vi "Plot.vi"(5 "dev-Var data":dbl[](array[numeric]), 7 "Selected Variables":string[][](array[string])=[["EnergyMeter", "Channel1", "amp1", "32"], ["EnergyMeter", "Channel2", "amp2", "25"]], 9 "Currently selected items":i32[](array[numeric])) -> (4 "Plot Data":dbl[](array[numeric]))   [LabVIEW 2020]
doc: "This vi parse the configuration file data into requires to plot short term and long term plot\n[input]\n1. Selected variables\n2. Selected indices\n3. Data from TCP connection\n[output]\n1. Plot names for plot legend\n2. Plot data"
uses:
  <userlib>/_OpenG.lib/array/array.llb/Index 1D Array Elements (DBL)__ogtk.vi
panel:
  out "References":string[](array[string])
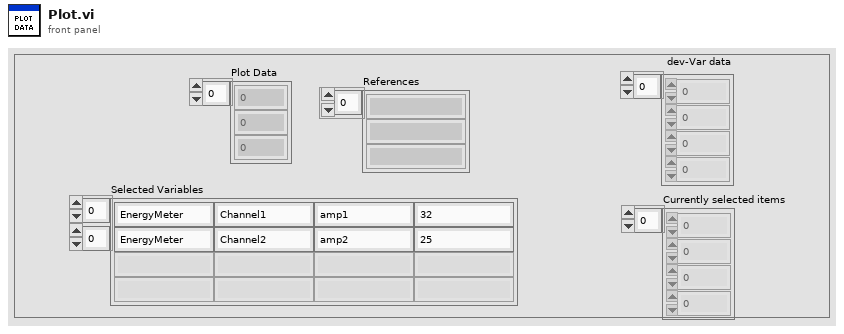
[diagram p1: front panel]
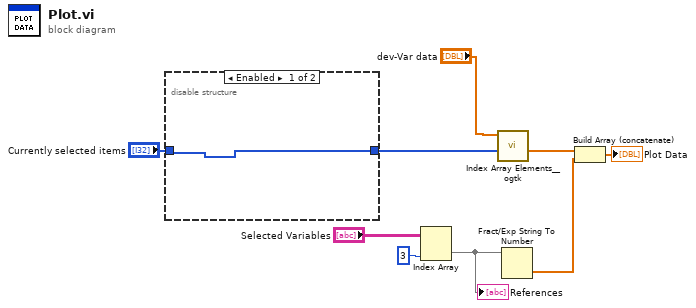
[diagram p0: block diagram]
diagram:
  n1 = disable-structure shown="Enabled" {
    disable-tunnel: "Currently selected items" -> [w10 w11]
    disable-tunnel: [w10 w11] -> w2
    frame Enabled {
    }
    frame Disabled {
    }
  }
  n2 = Index Array(array="Selected Variables", index (col)=3 ("disabled index (col)")) -> (element=w7:string[])  [unwired: 1 in]
  "References" <- w7
  n3 = call-poly <userlib>:"Index Array Elements__ogtk.vi"("indices"=w2, "array"="dev-Var data") -> ("elements"=w6:dbl[])  [unwired: 9 in]
  n4 = Fract/Exp String To Number(string=w7) -> (number=w4:dbl[])  [unwired: 3 in, 1 out]
  n5 = Build Array (concatenate)(w6, w4) -> (→"Plot Data":dbl[])
